vi "PDCConvertRecRate.vi"(10 "RecRateValue":u16, 11 "RecRateList":string[](array[string])) -> (3 "RecRate":u32)   [LabVIEW 2015]
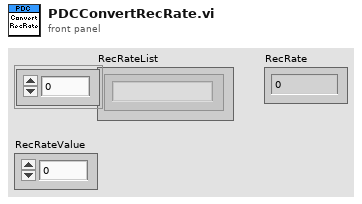
[diagram p1: front panel]
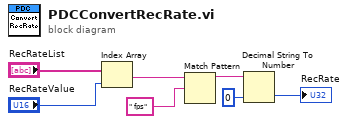
[diagram p0: block diagram]
diagram:
  n1 = Index Array(array="RecRateList", index="RecRateValue") -> (element=w4:string)
  n2 = Match Pattern(string=w4, regular expression=" fps") -> (before substring=w2:string)  [unwired: 4 out]
  n3 = Decimal String To Number(string=w2, default (0L)=u32 0 ("デフォルト (0 I32)")) -> (number=→"RecRate":u32)  [unwired: 2 out]
